vi "Obtener_valor_ADC.vi"(11 "ADC Response":string) -> (3 "Valor_ADC":dbl)   [LabVIEW 2019]
uses:
  <vilib>/regexp/Match Regular Expression.xnode
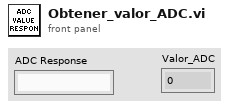
[diagram p1: front panel]
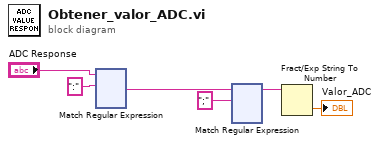
[diagram p0: block diagram]
diagram:
  n1 = xnode "Match Regular Expression"("input string"="ADC Response", "regular expression"=":") -> ("after match"=w4:string)  [unwired: 4 in, 4 out]
  n2 = xnode "Match Regular Expression"("input string"=w4, "regular expression"=";") -> ("before match"=w2:string)  [unwired: 4 in, 4 out]
  n3 = Fract/Exp String To Number(string=w2) -> (number=→"Valor_ADC":dbl)  [unwired: 3 in, 1 out]
